vi "xinput.vi"(11 "file path (dialog if empty)":path) -> (3 "Dynamic Data":dynamicdata(waveform))   [LabVIEW 2011]
uses:
  <vilib>/Utility/file.llb/Read From Spreadsheet File (DBL).vi
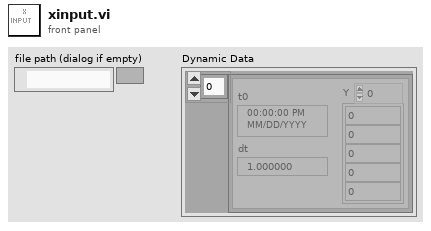
[diagram p1: front panel]
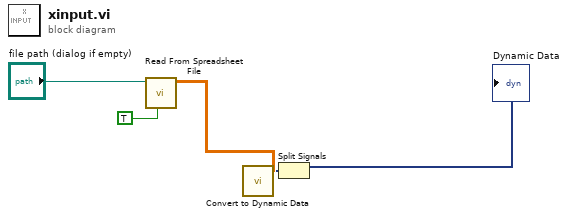
[diagram p0: block diagram]
diagram:
  n1 = call-poly <vilib>:"Read From Spreadsheet File.vi"("transpose (no:F)"=TRUE, "file path (dialog if empty)"="file path (dialog if empty)") -> ("all rows"=w3:dbl[][])  [unwired: 5 in, 4 out]
  n2 = call "Convert to Dynamic Data"("2D Array"=w3) -> ("Dynamic Data Type"=w2:dynamicdata)  [unwired: 3 in]
  n3 = Split Signals(w2) -> (→"Dynamic Data":dynamicdata)  [unwired: 2 in, 1 out]
